vi "CNT Set Value.vi"(9 "pCntValues":u32[](array[numeric])=[0, 0, 0, 0, 0, 0, 0, 0], 10 "ChannelMask":u8, 11 "DevHandle":i32) -> (1 "pCntValues out":u32[](array[numeric]), 3 "function return":i32)   [LabVIEW 2010, in "usb2cnt.lvlib"]
doc: "int WINAPI CNT_SetValue(int DevHandle, unsigned char ChannelMask,unsigned int *pCntValues);"
uses:
  usb2cnt.lvlib
  USB2XXX.dll
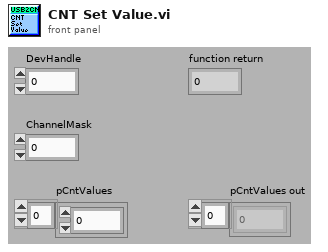
[diagram p1: front panel]
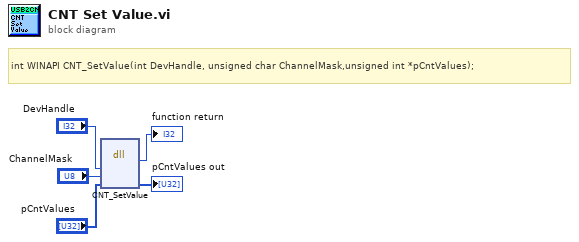
[diagram p0: block diagram]
diagram:
  # "int WINAPI CNT_SetValue(int DevHandle, unsigned char ChannelMask,unsigned int *pCntValues);"
  n1 = dll-call lib="G:/OtherWork/USB2XXX_Example/trunk/Labview/PublicFiles/USB2XXX.*" fn="CNT_SetValue"("DevHandle"="DevHandle", "ChannelMask"="ChannelMask", "pCntValues"="pCntValues") -> (→"function return":i32, "pCntValues"=→"pCntValues out":u32[])  [unwired: 5 in, 2 out]
